vi "NodosPropiedad_Graficas.vi"() -> ()   [LabVIEW 2020]
uses:
  <vilib>/numeric/Random Number (Range) DBL.vi
panel:
  out "Temperature":cluster{"number":dbl, "High Limit":dbl}(graph)
  out "Date and Time":string
  out "Out of Range":bool
  in  "High Limit":dbl
  in  "Sample Rate (ms)":u32
  out "Points Acqured":i32
  in  "Points to Acquare":i32
  in  "Stop":bool
  # "Equipo Dinamita \"RochaLovers\""
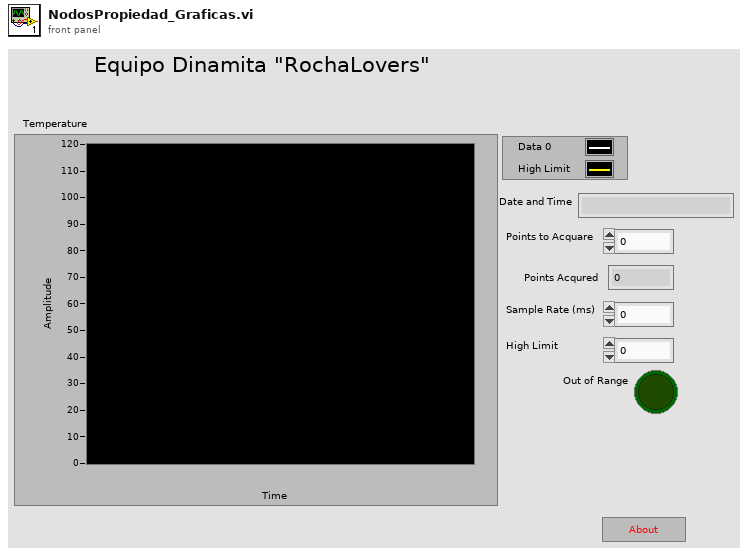
[diagram p1: front panel]
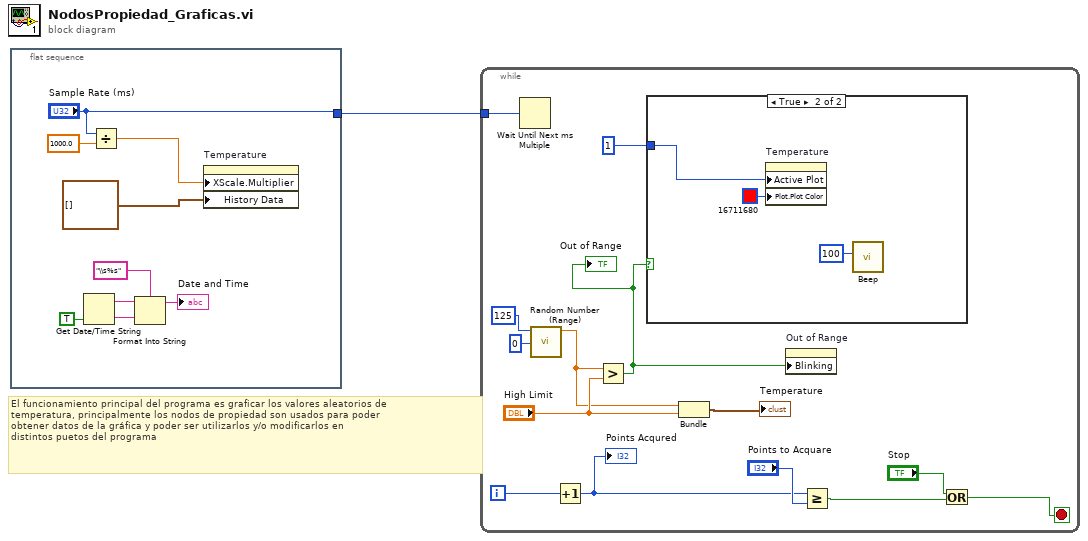
[diagram p0: block diagram]
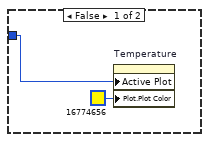
[diagram p2: hidden frame]
diagram:
  # "El funcionamiento principal del programa es graficar los valores aleatorios de \ntemperatura, principalmente los nodos de propiedad son usados para poder\nobtener datos de la gráfica y poder ser utilizarlos y/o modificarlos en \ndistintos puetos del programa"
  n1 = flat-sequence {
    tunnel: ["Sample Rate (ms)"] -> w1
    frame #0 {
      n2 = Get Date/Time String(want seconds? (F)=TRUE) -> (date string=w7:string, time string=w8:string)  [unwired: 2 in]
      n3 = Divide(x="Sample Rate (ms)", y=1000.0) -> (x/y=w5:dbl)
      n4 = Format Into String(format string="\\s%s", initial string=w7, w8) -> (resulting string=→"Date and Time":string)  [unwired: 1 in, 1 out]
      n5 = property on="Temperature" class="WFChart (strict)"("XScale.Multiplier"=w5, "History Data"=cluster{"number":dbl, "High Limit":dbl}[] []) -> ()  [unwired: 2 in, 2 out]
    }
  }
  n6 = while {
    tunnel: w1 -> [w24]
    i -> [w18]
    stop <- w14 stop-if-true
    n7 = Wait Until Next ms Multiple(millisecond multiple=w24) -> ()  [unwired: 1 out]
    n8 = call-poly <vilib>:"Random Number (Range).vi"("lower bound (0)"=u64 0, "upper bound (100)"=u64 125) -> ("number"=w20:dbl)  [unwired: 9 in]
    n9 = Increment(x=w18) -> (x+1=w11:i32)
    "Points Acqured" <- w11
    n10 = Greater?(x=w20, y="High Limit") -> (0:w13:bool)
    "Out of Range" <- w13
    n11 = case shown="True" w13 {
      tunnel: 1 -> [w26 w29]
      frame False {
        n12 = property on="Temperature" class="WFChart (strict)"("Active Plot"=w26, "Plot.Plot Color"=u32 16774656) -> ()  [unwired: 2 in, 2 out]
      }
      frame True {
        n13 = property on="Temperature" class="WFChart (strict)"("Active Plot"=w29, "Plot.Plot Color"=u32 16711680) -> ()  [unwired: 2 in, 2 out]
        n14 = call <vilib>:"Beep.vi"("duration (msec)"=u32 100) -> ()  [unwired: 11 in]
      }
    }
    n15 = Bundle("number"=w20, "High Limit"="High Limit") -> (→"Temperature":cluster{"number":dbl, "High Limit":dbl})  [unwired: 1 in]
    n16 = property on="Out of Range" class="Bool (strict)"("Blinking"=w13) -> ()  [unwired: 2 in, 2 out]
    n17 = Greater Or Equal?(x=w11, y="Points to Acquare") -> (x >= y?=w16:bool)
    n18 = Or(x="Stop", y=w16) -> (x .or. y?=w14:bool)
  }
